vi "Reserve Climb.vi"(4 "Reset Climb Encoder":bool, 6 "Reset Climb State":bool, 7 "Description":string="Reserve", 8 "Command Info":T1, 10 "Command Name":string) -> (0 "Command Info":T1)   [LabVIEW 2020]
uses:
  <vilib>/Rock Robotics/WPI/Framework/Command Status Info.ctl
  <vilib>/Rock Robotics/WPI/Framework/Completion Status.ctl
  <vilib>/Rock Robotics/WPI/Framework/Completion Notifier.ctl
  Implementation/Climb Setpoints.ctl
  Implementation/Climb Operations.ctl
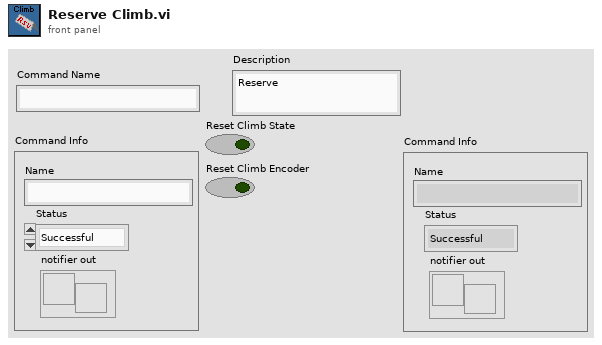
[diagram p1: front panel]
types:
  T1 = typedef "Command Status Info.ctl" = cluster{"Name":string, "Status":T2, "notifier out":T3}
  T2 = typedef "Completion Status.ctl" = enum16{"Successful", "Aborted", "Incomplete"}
  T3 = typedef "Completion Notifier.ctl" = refnum<notifier>
  T4 = typedef "Climb Setpoints.ctl" = cluster{"Operation":T5, "Extension Setpoint":dbl, "Pivot Setpoint":dbl, "Reset Climb State":bool, "Reset Climb Encoder":bool}
  T5 = typedef "Climb Operations.ctl" = enum16{"Reserve", "Read Current", "Immediate", "Auto Climb: Next Stage"}
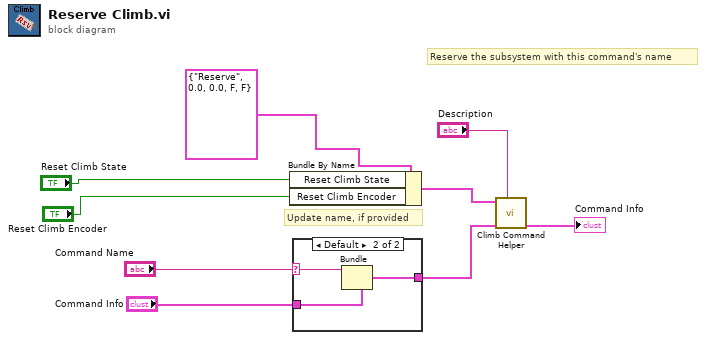
[diagram p0: block diagram]
diagram:
  # "Update name, if provided"
  # "Reserve the subsystem with this command's name"
  n1 = Bundle By Name(cluster=T4 {"Operation"=enum."Reserve", "Extension Setpoint"=0.0, "Pivot Setpoint"=0.0, "Reset Climb State"=FALSE, "Reset Climb Encoder"=FALSE} ("SubSystem Data"), "Reset Climb State"="Reset Climb State", "Reset Climb Encoder"="Reset Climb Encoder") -> (w1:T4)
  n2 = case shown="Default" "Command Name" {
    selector: "Command Name" -> [_ w11]
    tunnel: "Command Info" -> [w10 w13]
    tunnel: [w10 w12] -> w6
    frame "" {
    }
    frame Default {
      n3 = Bundle(cluster=w13, "Name"=w11) -> (w12:T1)  [unwired: 2 in]
    }
  }
  n4 = call "Climb Command Helper.vi"("Description"="Description", "Command Info In"=w6, "SubSystem Data"=w1) -> ("Command Info Out"=→"Command Info":T1)  [unwired: 6 in, 2 out]
